vi "AO Configure Timing.vi"(8 "error in (no error)":errorcluster, 10 "Params":variant, 11 "NI Analog Output in":refnum<class "NI Analog Output.lvclass">) -> (0 "error out":errorcluster, 3 "NI Analog Output out":refnum<class "NI Analog Output.lvclass">)   [LabVIEW 2020, in "NI DAQmx.lvlib" / "NI Analog Output.lvclass"]
uses:
  NI Analog Output.lvclass
  D:/WSGitHub/RTFWK/Realization/NI DAQmx Base/NI DAQmx Base.lvclass
  TypeDefs/Timing Config.ctl
  <vilib>/DAQmx/configure/timing.llb/DAQmx Timing (Sample Clock).vi
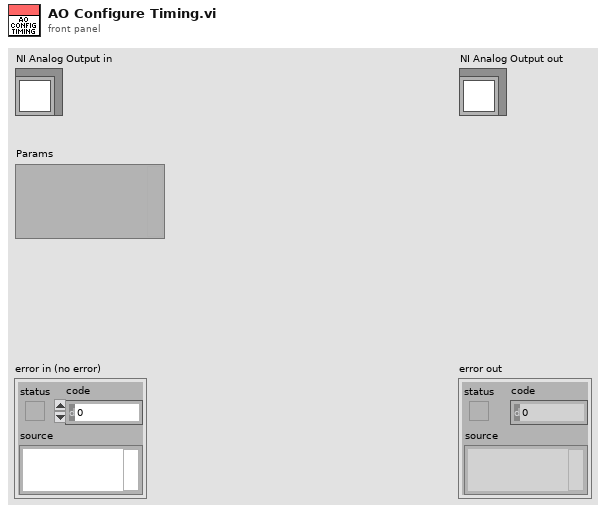
[diagram p1: front panel]
types:
  T1 = typedef "Timing Config.ctl" = cluster{"sample mode":i32, "samples per channel":i32, "rate":dbl, "source":string, "active edge":i32}
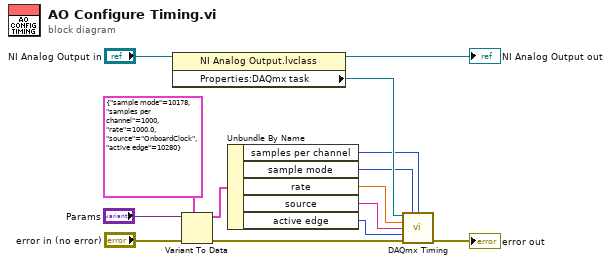
[diagram p0: block diagram]
diagram:
  n1 = property class="NI Analog Output.lvclass"(reference="NI Analog Output in") -> (reference out=→"NI Analog Output out":refnum<class "NI Analog Output.lvclass">, "Properties:DAQmx task"=w8:refnum<k21>)  [unwired: 1 in, 1 out]
  n2 = Variant To Data(error in="error in (no error)", type=T1 {"sample mode"=10178, "samples per channel"=1000, "rate"=1000.0, "source"="OnboardClock", "active edge"=10280}, Variant="Params") -> (data=w6:T1, error out=w10:errorcluster)
  n3 = Unbundle By Name(w6) -> ("samples per channel"=w1:i32, "sample mode"=w2:i32, "rate"=w5:dbl, "source"=w4:string, "active edge"=w3:i32)
  n4 = call-poly <vilib>:"DAQmx Timing.vi"("task/channels in"=w8, "sample mode"=w2, "samples per channel"=w1, "rate"=w5, "source"=w4, "active edge"=w3, "error in"=w10) -> ("error out"=→"error out":errorcluster)  [unwired: 7 in, 1 out]
